vi "tlc_Timing Stop Module.vi"(7 "Command (Stop)":T1=enum."Stop", 8 "error in (no error)":errorcluster, 10 "Play Structure Names":T2) -> (0 "error out":errorcluster)   [LabVIEW 2018]
uses:
  Controls/Play Structure Names.ctl
  tlc_Timing Stop Module Control.ctl
panel:
  # "Input"
  # "Output"
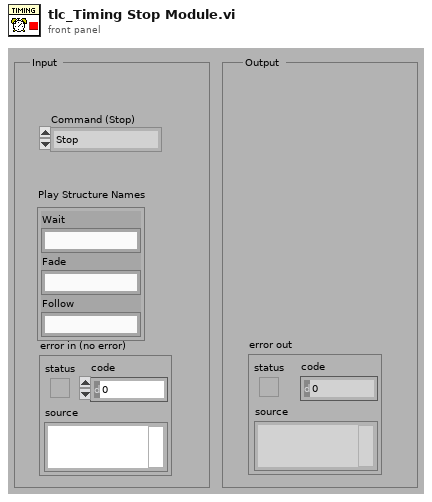
[diagram p1: front panel]
types:
  T1 = typedef "tlc_Timing Stop Module Control.ctl" = enum16{"Intialize", "Stop"}
  T2 = typedef "Play Structure Names.ctl" = cluster{"Wait":string, "Fade":string, "Follow":string}
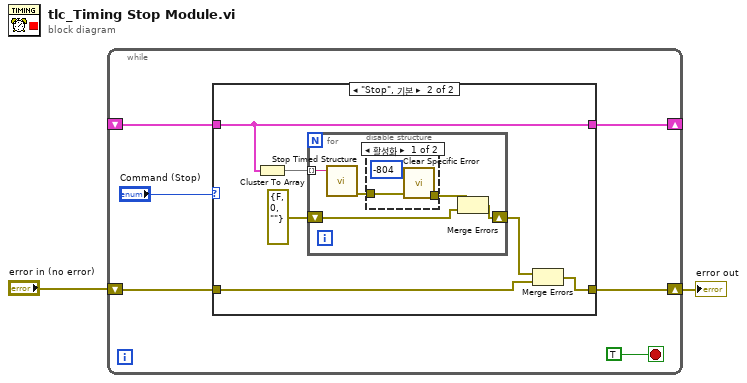
[diagram p0: block diagram]
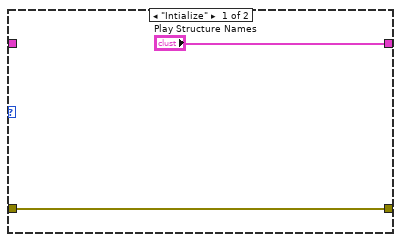
[diagram p2: hidden frame]
diagram:
  n1 = while {
    shift-right: [w6] -> _
    shift-left: _ -> [w5]
    shift-right: [w3] -> w1
    shift-left: "error in (no error)" -> [w4]
    stop <- TRUE stop-if-true
    n2 = case shown="\"Stop\", 기본" "Command (Stop)" {
      tunnel: ["Play Structure Names" w16] -> w6
      tunnel: w5 -> [_ w16]
      tunnel: w4 -> [w9 w12]
      tunnel: [w9 w11] -> w3
      frame "Intialize" {
      }
      frame "Stop", Default {
        n3 = Cluster To Array(cluster=w16) -> (array=w15:string[])
        n4 = for {
          tunnel: w15 -> [w21] mode=indexing
          shift-right: [w18] -> w13
          shift-left: errorcluster {"status"=FALSE, "code"=0, "source"=""} ("error out") -> [w17]
          n5 = call <vilib>:"Stop Timed Structure.vi"("name"=w21) -> ("error out"=w20:errorcluster)  [unwired: 10 in]
          n6 = disable-structure shown="활성화" {
            disable-tunnel: w20 -> [w24 w25]
            disable-tunnel: [w22 w25] -> w19
            frame Enabled {
              n7 = call "Clear Specific Error.vi"("error in (no error)"=w24, "Code"=-804) -> ("error out"=w22:errorcluster)  [unwired: 5 in]
            }
            frame Disabled {
            }
          }
          n8 = Merge Errors(w19, w17) -> (w18:errorcluster)
        }
        n9 = Merge Errors(w13, w12) -> (w11:errorcluster)
      }
    }
  }
  "error out" <- w1
